vi "Create ImageList.vi"(8 "error in (no error)":errorcluster caption="错误输入（无错误）", 10 "ImgPath":path[](array[path]), 11 "StatusStripClass 输入":refnum<class "StatusStripClass.lvclass"> caption="DNL_LabVIEW Object in") -> (0 "error out":errorcluster caption="错误输出", 3 "StatusStripClass 输出":refnum<class "StatusStripClass.lvclass"> caption="DNL_LabVIEW Object out")   [LabVIEW 2013, in "StatusStripClass.lvclass"]
uses:
  StatusStripClass.lvclass
  StatusStripClass.lvclass/StatusStripClass.ctl
  System.Windows.Forms
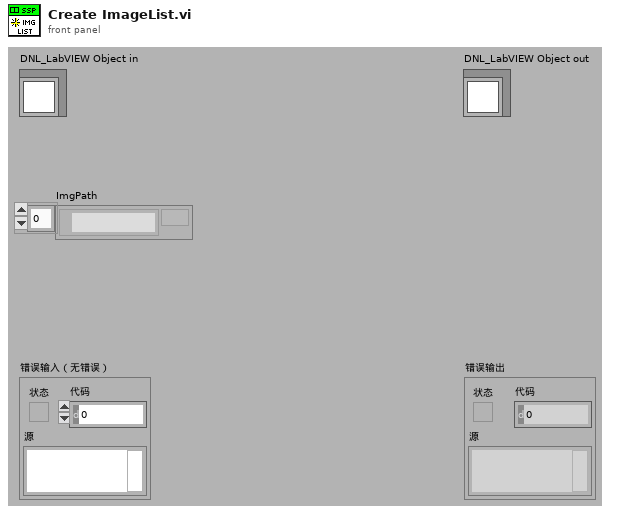
[diagram p1: front panel]
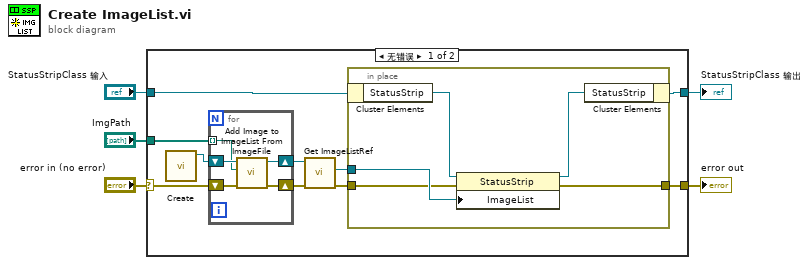
[diagram p0: block diagram]
diagram:
  n1 = case shown="无错误" "error in (no error)" {
    selector: "error in (no error)" -> [w12 w27]
    tunnel: [w7 w27] -> w4
    tunnel: [w6 w26] -> w2
    tunnel: "StatusStripClass 输入" -> [w15 w26]
    tunnel: "ImgPath" -> [w14 _]
    frame No Error {
      n2 = call "Create.vi"() -> ("ImageListClass 输出"=w13:refnum<class "ImageListClass.lvclass">)  [unwired: 10 in, 1 out]
      n3 = for {
        tunnel: w14 -> [w16] mode=indexing
        shift-right: [w19] -> w11
        shift-left: w13 -> [w20]
        shift-right: [w17] -> w10
        shift-left: w12 -> [w18]
        n4 = call "Add Image to ImageList From ImageFile.vi"("error in (no error)"=w18, "Path"=w16, "ImageListClass 输入"=w20) -> ("error out"=w17:errorcluster, "ImageListClass 输出"=w19:refnum<class "ImageListClass.lvclass">)  [unwired: 7 in]
      }
      n5 = call "Get ImageListRef.vi"("error in (no error)"=w10, "ImageListClass 输入"=w11) -> ("error out"=w8:errorcluster, "ImageList"=w9:refnum<k24>)  [unwired: 7 in, 1 out]
      n6 = in-place {
        in-place-border: w9 -> [w23]
        in-place-border: w8 -> [w22]
        in-place-border: [w21] -> w7
        n7 = in-place-cluster #1(w15) -> ("StatusStrip"=w25:refnum<k24>)
        n8 = property class="StatusStrip"(reference=w25, error in=w22, "ImageList"=w23) -> (reference out=w24:refnum<k24>, error out=w21:errorcluster)
        n9 = in-place-cluster #1("StatusStrip"=w24) -> (w6:refnum<class "StatusStripClass.lvclass">)
      }
    }
    frame Error {
    }
  }
  "error out" <- w4
  "StatusStripClass 输出" <- w2
